vi "Focus Standard Variation.vi"(8 "error in":errorcluster, 9 "Scan Increments":dbl=0.01 format="%#_13g", 10 "Component":T1, 11 "Gantry In":refnum<k24>) -> (0 "error out":errorcluster, 2 "max value":dbl, 3 "Gantry Out":refnum<k24>)   [LabVIEW 2021, in "Component Tray.lvclass"]
uses:
  Component/Component Tray.lvclass
  C:/Program Files (x86)/Aerotech/A3200/LabVIEW/2010/Bin/Aerotech.A3200.dll
  Program Files (x86)/Aerotech/A3200/LabVIEW/2010/Bin/Aerotech.A3200.dll
  Component/Find Component.ctl
  Controller/Camera/Machine Vision.ctl
  Controller/Motion/A3200/A3200.lvclass
  Controller/Camera/Camera.lvclass
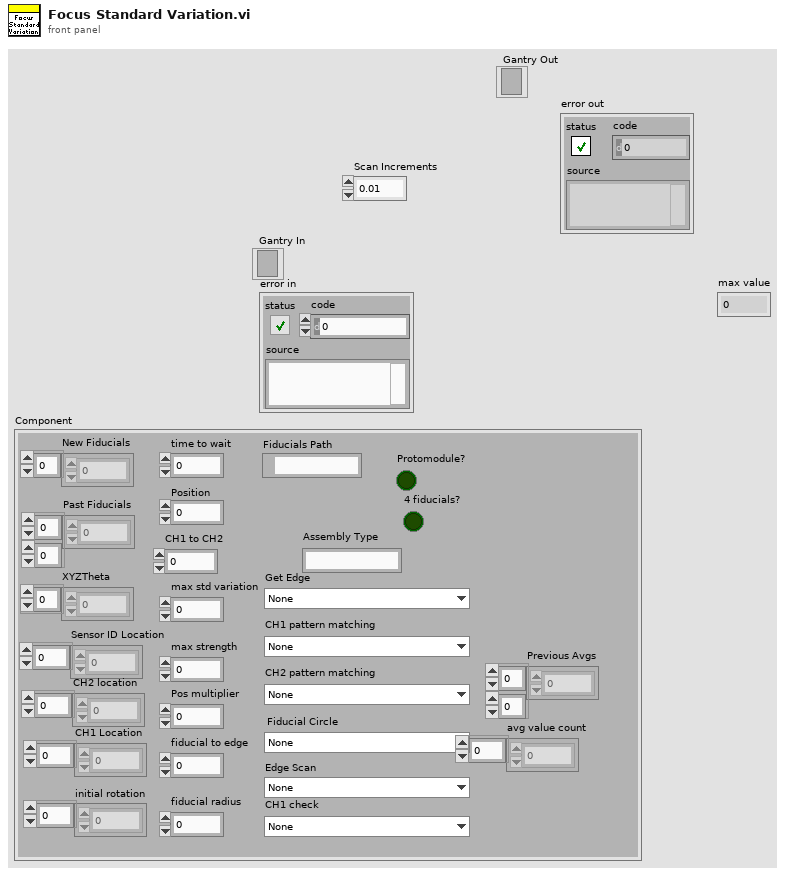
[diagram p1: front panel]
types:
  T1 = typedef "Component Tray.lvclass/Find Component.ctl" = cluster{"New Fiducials":dbl[], "Past Fiducials":dbl[][], "XYZTheta":dbl[], "Fiducials Path":path, "Position":i32, "CH1 Location":dbl[], "Sensor ID Location":dbl[], "initial rotation":dbl[], "CH2 location":dbl[], "max std variation":dbl, "max strength":dbl, "CH2 pattern matching":T2, "Fiducial Circle":T2, "Get Edge":T2, "Pos multiplier":dbl, "time to wait":u32, "fiducial to edge":dbl, "Protomodule?":bool, "Assembly Type":string, "CH1 to CH2":dbl, "Tray Number":string, "fiducial radius":dbl, "4 fiducials?":bool, "CH1 check":T2, "Edge Scan":T2, "CH1 pattern matching":T2, "Sensor Thickness":dbl, "Previous Avgs":dbl[][], "avg value count":dbl[]}
  T2 = typedef "Camera.lvclass/Machine Vision.ctl" = enum16{"None", "Assembly Tray Circle", "Assembly Tray Fiducial", "Partial Hexaboard", "sensor edge init", "HB edge init", "sensor edge pos1", "sensor edge pos2", "HB edge pos1", "HB edge pos2", "Sensor CH1-2", "HB CH1", "HB CH2", "V3 Sensor Circle", "Hexaboard Circle", "sensor CH1 check", "HB CH1 check ", "sensor ID"}
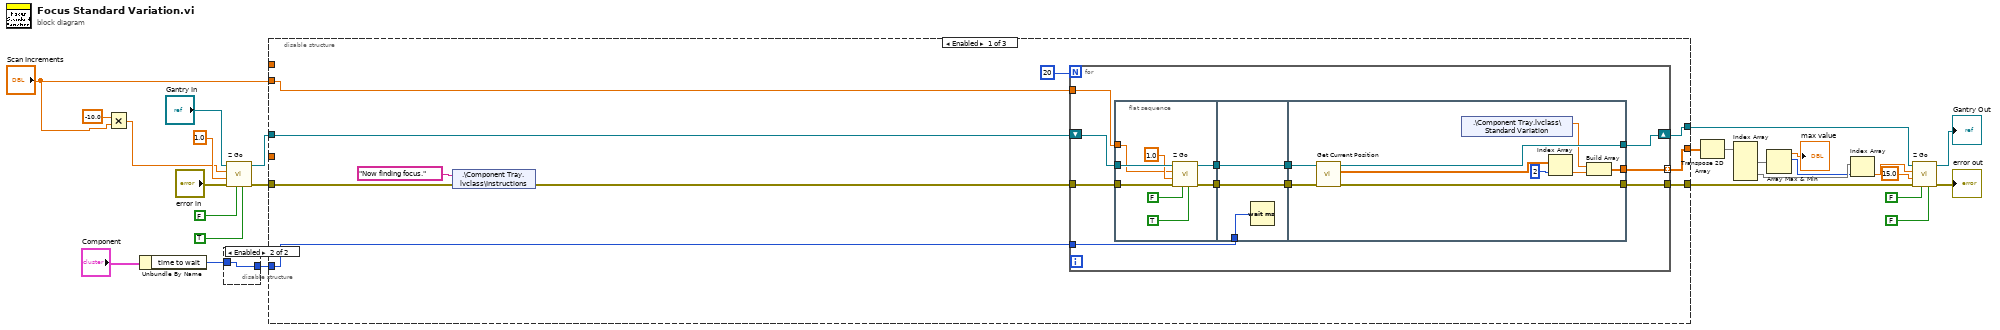
[diagram p0: block diagram]
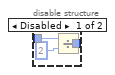
[diagram p2: hidden frame]
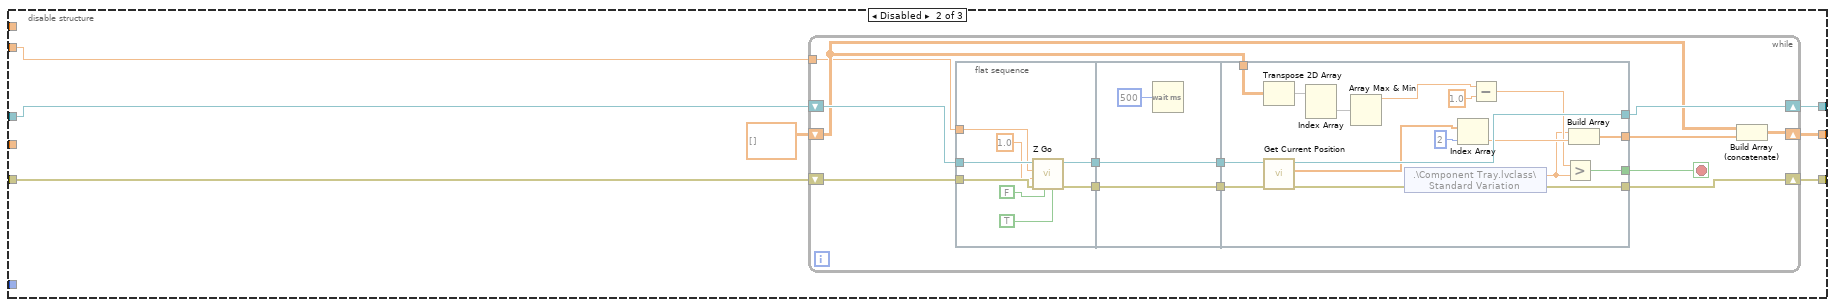
[diagram p3: hidden frame]
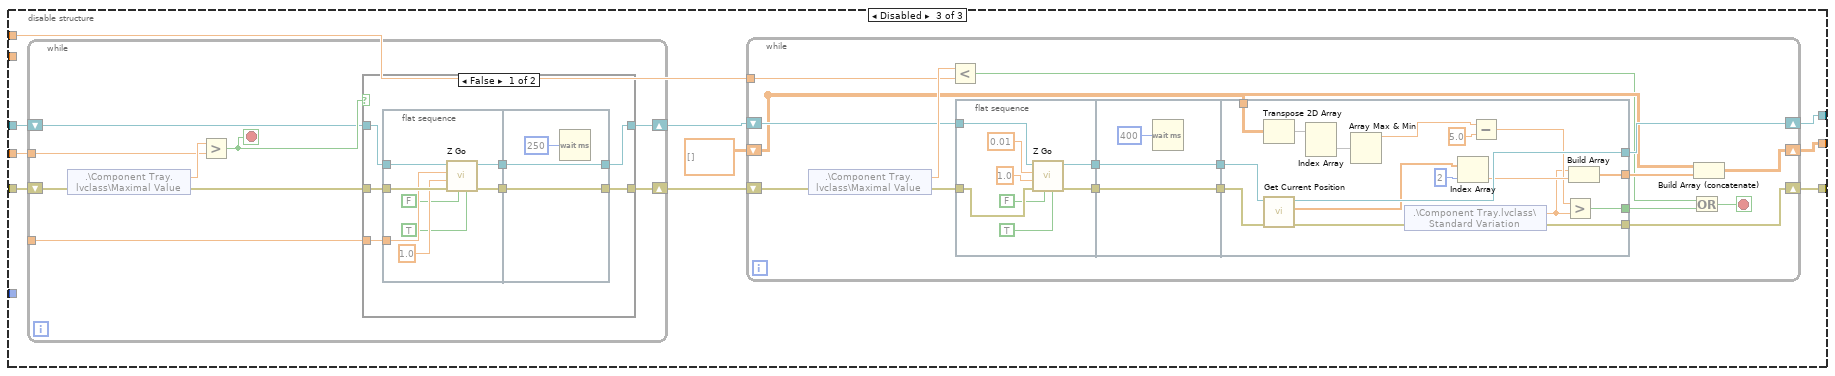
[diagram p4: hidden frame]
diagram:
  n1 = Multiply(x=-10.0, y="Scan Increments") -> (x*y=w4:dbl)
  n2 = Unbundle By Name("Component") -> ("time to wait"=w2:u32)
  n3 = disable-structure shown="Enabled" {
    disable-tunnel: w2 -> [w30 w31]
    disable-tunnel: [w28 w31] -> w1
    frame Disabled {
      n4 = Divide(x=w30, y=u32 2) -> (x/y=w28:dbl)
    }
    frame Enabled {
    }
  }
  n5 = call "Z Go.vi"("Increment"=TRUE, "Return Immediately"=FALSE ("Increment"), "error in (no error)"="error in", "Speed In"=1.0 ("Speed"), "Position In"=w4, "Gantry In"="Gantry In") -> ("error out"=w9:errorcluster, "Gantry Out"=w10:refnum<k24>)  [unwired: 2 in, 2 out]
  n6 = disable-structure shown="Enabled" {
    disable-tunnel: [w41 w75 w124] -> w24
    disable-tunnel: [w40 w76 w125] -> w21
    disable-tunnel: [w39 w77 w127] -> w20
    disable-tunnel: w10 -> [w38 w79 w130]
    disable-tunnel: w9 -> [w35 w78 w129]
    disable-tunnel: _ -> [_ _ w122]
    disable-tunnel: _ -> [_ _ w121]
    disable-tunnel: "Scan Increments" -> [w37 w73 _]
    disable-tunnel: w1 -> [w32 _ _]
    frame Enabled {
      n7 = shared-variable ".\\Component Tray.lvclass\\Instructions"("Now finding focus." ("Instructions"), error in=w35) -> (error out=w34:errorcluster)
      n8 = for {
        N: 20 -> [_]
        tunnel: [w50] -> w41 mode=indexing
        tunnel: w34 -> [w49]
        tunnel: [w48] -> w39
        shift-right: [w51] -> w40
        shift-left: w38 -> [w52]
        tunnel: w37 -> [w43]
        tunnel: w32 -> [w42]
        n9 = flat-sequence {
          tunnel: w52 -> [w60]
          tunnel: [w59] -> w47
          tunnel: w49 -> [w58]
          tunnel: [w57] -> w45
          tunnel: w43 -> [w55]
          tunnel: w47 -> [w63]
          tunnel: [w63] -> w46
          tunnel: w45 -> [w62]
          tunnel: [w62] -> w44
          tunnel: w42 -> [w61]
          tunnel: w46 -> [w72]
          tunnel: [w71] -> w51
          tunnel: [w70] -> w50
          tunnel: w44 -> [w69]
          tunnel: [w68] -> w48
          frame #0 {
            n10 = call "Z Go.vi"("Increment"=TRUE, "Return Immediately"=FALSE ("Increment"), "error in (no error)"=w58, "Speed In"=1.0 ("Speed"), "Position In"=w55, "Gantry In"=w60) -> ("error out"=w57:errorcluster, "Gantry Out"=w59:refnum<k24>)  [unwired: 2 in, 2 out]
          }
          frame #1 {
            n11 = Wait (ms)(milliseconds to wait=w61) -> ()  [unwired: 1 out]
          }
          frame #2 {
            n12 = call "Get Current Position.vi"("error in (no error)"=w69, "Gantry In"=w72) -> ("error out"=w68:errorcluster, "XYZTheta Out"=w67:dbl[], "Gantry Out"=w71:refnum<k24>)  [unwired: 7 in]
            n13 = shared-variable ".\\Component Tray.lvclass\\Standard Variation"() -> (w64:sgl)  [unwired: 1 in, 1 out]
            n14 = Index Array(array=w67, index=2) -> (element=w65:dbl)
            n15 = Build Array(w64, w65) -> (w70:dbl[])
          }
        }
      }
    }
    frame Disabled {
      n16 = while {
        shift-right: [w84] -> w75
        shift-left: dbl[][] [] -> [w83]
        shift-right: [w90] -> w76
        shift-left: w79 -> [w91]
        shift-right: [w92] -> w77
        shift-left: w78 -> [w81]
        tunnel: w73 -> [w80]
        stop <- w82 stop-if-true
        n17 = flat-sequence {
          tunnel: w91 -> [w100]
          tunnel: [w99] -> w89
          tunnel: w81 -> [w98]
          tunnel: [w97] -> w88
          tunnel: w80 -> [w93]
          tunnel: w89 -> [w103]
          tunnel: [w103] -> w87
          tunnel: w88 -> [w102]
          tunnel: [w102] -> w86
          tunnel: w87 -> [w120]
          tunnel: [w119] -> w90
          tunnel: [w118] -> w85
          tunnel: w86 -> [w114]
          tunnel: [w112] -> w92
          tunnel: w83 -> [w111]
          tunnel: [w104] -> w82
          frame #0 {
            n18 = call "Z Go.vi"("Increment"=TRUE, "Return Immediately"=FALSE ("Increment"), "error in (no error)"=w98, "Speed In"=1.0 ("Speed"), "Position In"=w93, "Gantry In"=w100) -> ("error out"=w97:errorcluster, "Gantry Out"=w99:refnum<k24>)  [unwired: 2 in, 2 out]
          }
          frame #1 {
            n19 = Wait (ms)(milliseconds to wait=u32 500) -> ()  [unwired: 1 out]
          }
          frame #2 {
            n20 = Transpose 2D Array(2D array=w111) -> (transposed array=w110:dbl[][])
            n21 = call "Get Current Position.vi"("error in (no error)"=w114, "Gantry In"=w120) -> ("error out"=w113:errorcluster, "XYZTheta Out"=w117:dbl[], "Gantry Out"=w119:refnum<k24>)  [unwired: 7 in]
            n22 = Index Array(array=w110) -> (element=w109:dbl[])  [unwired: 2 in]
            n23 = Array Max & Min(array=w109) -> (max value=w108:dbl)  [unwired: 3 out]
            n24 = shared-variable ".\\Component Tray.lvclass\\Standard Variation"(error in=w113) -> (w105:sgl, error out=w112:errorcluster)
            n25 = Index Array(array=w117, index=2) -> (element=w115:dbl)
            n26 = Subtract(x=w108, y=1.0) -> (x-y=w106:dbl)
            n27 = Greater?(x=w106, y=w105) -> (0:w104:bool)
            n28 = Build Array(w105, w115) -> (w118:dbl[])
          }
        }
        n29 = Build Array (concatenate)(w83, w85) -> (w84:dbl[][])
      }
    }
    frame Disabled {
      n30 = while {
        shift-right: [w181] -> w126
        shift-left: w130 -> [w182]
        shift-right: [w180] -> w128
        shift-left: w129 -> [w178]
        tunnel: _ -> [w179]
        tunnel: w122 -> [w176]
        stop <- w183 stop-if-true
        n31 = shared-variable ".\\Component Tray.lvclass\\Maximal Value"(error in=w178) -> (w184:sgl, error out=w177:errorcluster)
        n32 = Greater?(x=w184, y=w176) -> (0:w183:bool)
        n33 = case shown="False" w183 {
          tunnel: w182 -> [w189 w204]
          tunnel: [w186 w204] -> w181
          tunnel: [w185 w203] -> w180
          tunnel: w177 -> [w188 w203]
          tunnel: w179 -> [w187 _]
          frame False {
            n34 = flat-sequence {
              tunnel: w189 -> [w199]
              tunnel: [w198] -> w191
              tunnel: w188 -> [w197]
              tunnel: [w196] -> w190
              tunnel: w187 -> [w194]
              tunnel: w191 -> [w201]
              tunnel: w190 -> [w200]
              tunnel: [w201] -> w186
              tunnel: [w200] -> w185
              frame #0 {
                n35 = call "Z Go.vi"("Increment"=TRUE, "Return Immediately"=FALSE ("Increment"), "error in (no error)"=w197, "Speed In"=1.0 ("Speed"), "Position In"=w194, "Gantry In"=w199) -> ("error out"=w196:errorcluster, "Gantry Out"=w198:refnum<k24>)  [unwired: 2 in, 2 out]
              }
              frame #1 {
                n36 = Wait (ms)(milliseconds to wait=u32 250) -> ()  [unwired: 1 out]
              }
            }
          }
          frame True {
          }
        }
      }
      n37 = while {
        shift-right: [w136] -> w124
        shift-left: dbl[][] [] -> [w134]
        tunnel: w121 -> [w135]
        shift-right: [w144] -> w125
        shift-left: w126 -> [w145]
        shift-right: [w146] -> w127
        shift-left: w128 -> [w143]
        stop <- w132 stop-if-true
        n38 = shared-variable ".\\Component Tray.lvclass\\Maximal Value"(error in=w143) -> (w147:sgl, error out=w142:errorcluster)
        n39 = Less?(x=w147, y=w135) -> (x < y?=w133:bool)
        n40 = flat-sequence {
          tunnel: w145 -> [w155]
          tunnel: [w154] -> w141
          tunnel: w142 -> [w153]
          tunnel: [w152] -> w140
          tunnel: w141 -> [w158]
          tunnel: [w158] -> w139
          tunnel: w140 -> [w157]
          tunnel: [w157] -> w138
          tunnel: w139 -> [w175]
          tunnel: [w174] -> w144
          tunnel: [w173] -> w137
          tunnel: w138 -> [w169]
          tunnel: [w167] -> w146
          tunnel: w134 -> [w166]
          tunnel: [w159] -> w131
          frame #0 {
            n41 = call "Z Go.vi"("Increment"=TRUE, "Return Immediately"=FALSE ("Increment"), "error in (no error)"=w153, "Speed In"=1.0 ("Speed"), "Position In"=0.01, "Gantry In"=w155) -> ("error out"=w152:errorcluster, "Gantry Out"=w154:refnum<k24>)  [unwired: 2 in, 2 out]
          }
          frame #1 {
            n42 = Wait (ms)(milliseconds to wait=u32 400) -> ()  [unwired: 1 out]
          }
          frame #2 {
            n43 = Transpose 2D Array(2D array=w166) -> (transposed array=w165:dbl[][])
            n44 = call "Get Current Position.vi"("error in (no error)"=w169, "Gantry In"=w175) -> ("error out"=w168:errorcluster, "XYZTheta Out"=w172:dbl[], "Gantry Out"=w174:refnum<k24>)  [unwired: 7 in]
            n45 = Index Array(array=w165) -> (element=w164:dbl[])  [unwired: 2 in]
            n46 = Array Max & Min(array=w164) -> (max value=w163:dbl)  [unwired: 3 out]
            n47 = shared-variable ".\\Component Tray.lvclass\\Standard Variation"(error in=w168) -> (w160:sgl, error out=w167:errorcluster)
            n48 = Index Array(array=w172, index=2) -> (element=w170:dbl)
            n49 = Subtract(x=w163, y=5.0) -> (x-y=w161:dbl)
            n50 = Greater?(x=w161, y=w160) -> (0:w159:bool)
            n51 = Build Array(w160, w170) -> (w173:dbl[])
          }
        }
        n52 = Or(x=w133, y=w131) -> (x .or. y?=w132:bool)
        n53 = Build Array (concatenate)(w134, w137) -> (w136:dbl[][])
      }
    }
  }
  n54 = Transpose 2D Array(2D array=w24) -> (transposed array=w14:dbl[][])
  n55 = Index Array(array=w14) -> (element #1=w11:dbl[], element #2=w13:dbl[])  [unwired: 4 in]
  n56 = Array Max & Min(array=w11) -> (max value=→"max value":dbl, max index (indices)=w12:i32)  [unwired: 2 out]
  n57 = Index Array(array=w13, index=w12) -> (element=w23:dbl)
  n58 = call "Z Go.vi"("Increment"=FALSE, "Return Immediately"=FALSE ("Increment"), "error in (no error)"=w20, "Speed In"=15.0 ("Speed"), "Position In"=w23, "Gantry In"=w21) -> ("error out"=→"error out":errorcluster, "Gantry Out"=→"Gantry Out":refnum<k24>)  [unwired: 2 in, 2 out]
